vi "Create Response Single Channel_Comparison.vi"(8 "error in (no error)":errorcluster, 10 "Properties":T1, 11 "Message refnum in":T2=18446744073709551615 format="%.0x") -> (0 "error out":errorcluster, 2 "Channel refnum out":T2=18446744073709551615 format="%.0x", 3 "Message refnum out":T2=18446744073709551615 format="%.0x")   [LabVIEW 2019, in "Scripting API.lvlib"]
uses:
  Scripting API.lvlib
  <vilib>/NI VeriStand/Custom Device API/Custom Device Item Ref.ctl
  <vilib>/NI VeriStand/Custom Device API/Custom Device API.lvlib
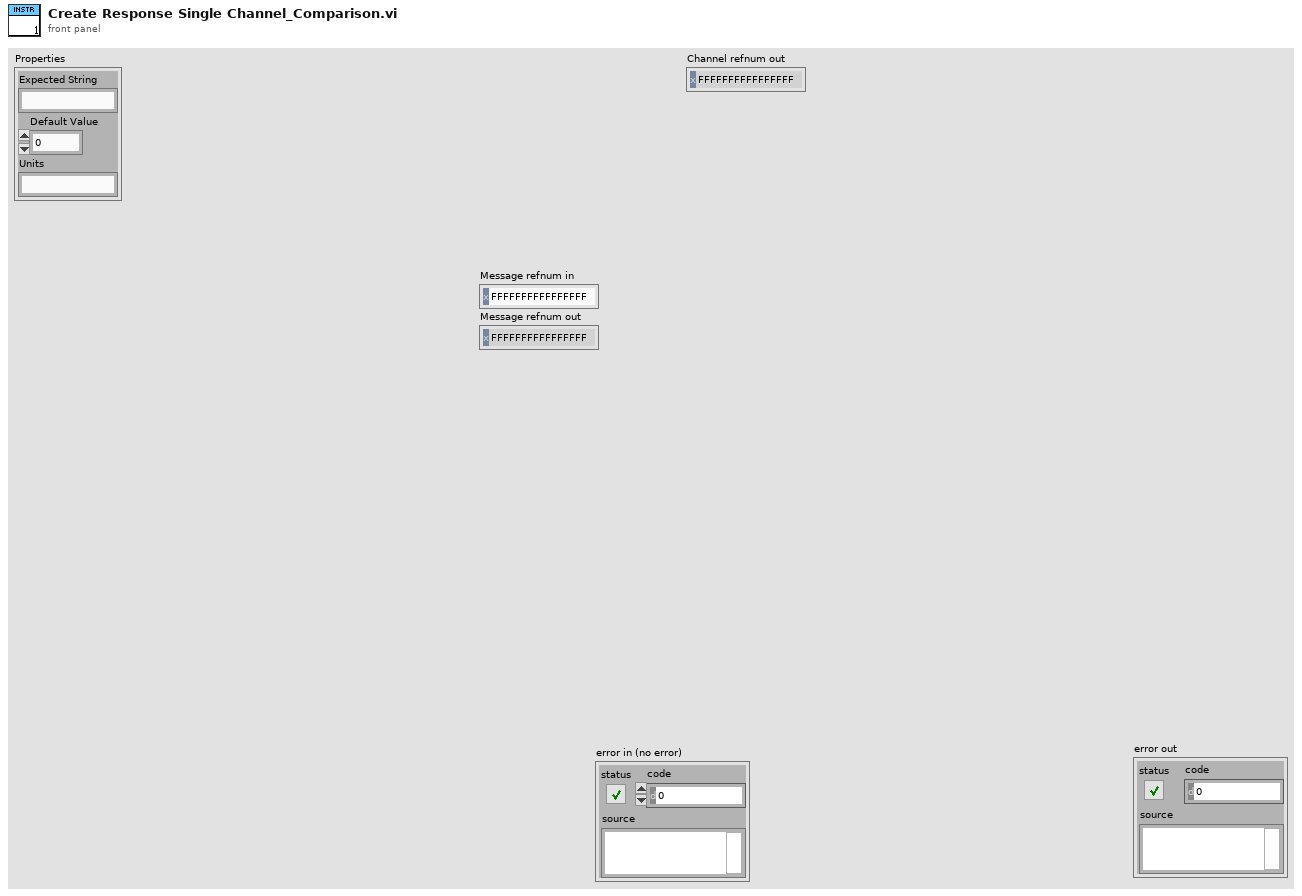
[diagram p1: front panel]
types:
  T1 = cluster{"Expected String":string, "Default Value":dbl, "Units":string}
  T2 = typedef "Custom Device API.lvlib/Custom Device Item Ref.ctl" = u64
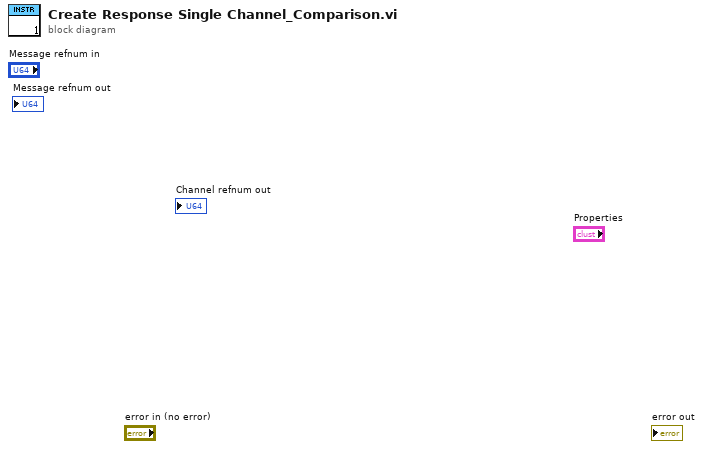
[diagram p0: block diagram]
diagram:
